vi "pickDefensiveTeam.vi"(0 "DefensiveTeam in":refnum<class "Ally.lvclass">, 1 "BallRef":refnum<class "Ball.lvclass">, 5 "KeeperTeam":refnum<class "Ally.lvclass">, 7 "OffensiveTeam":refnum<class "Ally.lvclass">, 9 "RobotRef in":refnum<class "Robot.lvclass">[](array[class]), 11 "error in (no error)":errorcluster, 12 "number_of_robots":i32, 13 "AllyTeamArray":T1[](array[typedef])) -> (4 "DefensiveTeam out":refnum<class "Ally.lvclass">, 8 "RobotRef":refnum<class "Robot.lvclass">[](array[class]), 15 "error out":errorcluster)   [LabVIEW 2023, in "Ally.lvclass"]
uses:
  Ally.lvclass
  Robot_class/Robot.lvclass
  Ball_class/Ball.lvclass
  Controls/AllyTeam.ctl
  Team_class/KeeperPlay.ctl
  Team_class/OffensivePlay.ctl
  Team_class/Team.lvclass/Team.ctl
  Robot_class/Robot.lvclass/Robot.ctl
  Utilities_class/Utilities.lvclass
  Robot_class/Read id.vi
  Team_class/Write RobotRef.vi
  Team_class/Read OffensivePlay.vi
  Team_class/Read RobotRef.vi
  Team_class/Read KeeperPlay.vi
  Team_class/Read DefensivePlay.vi
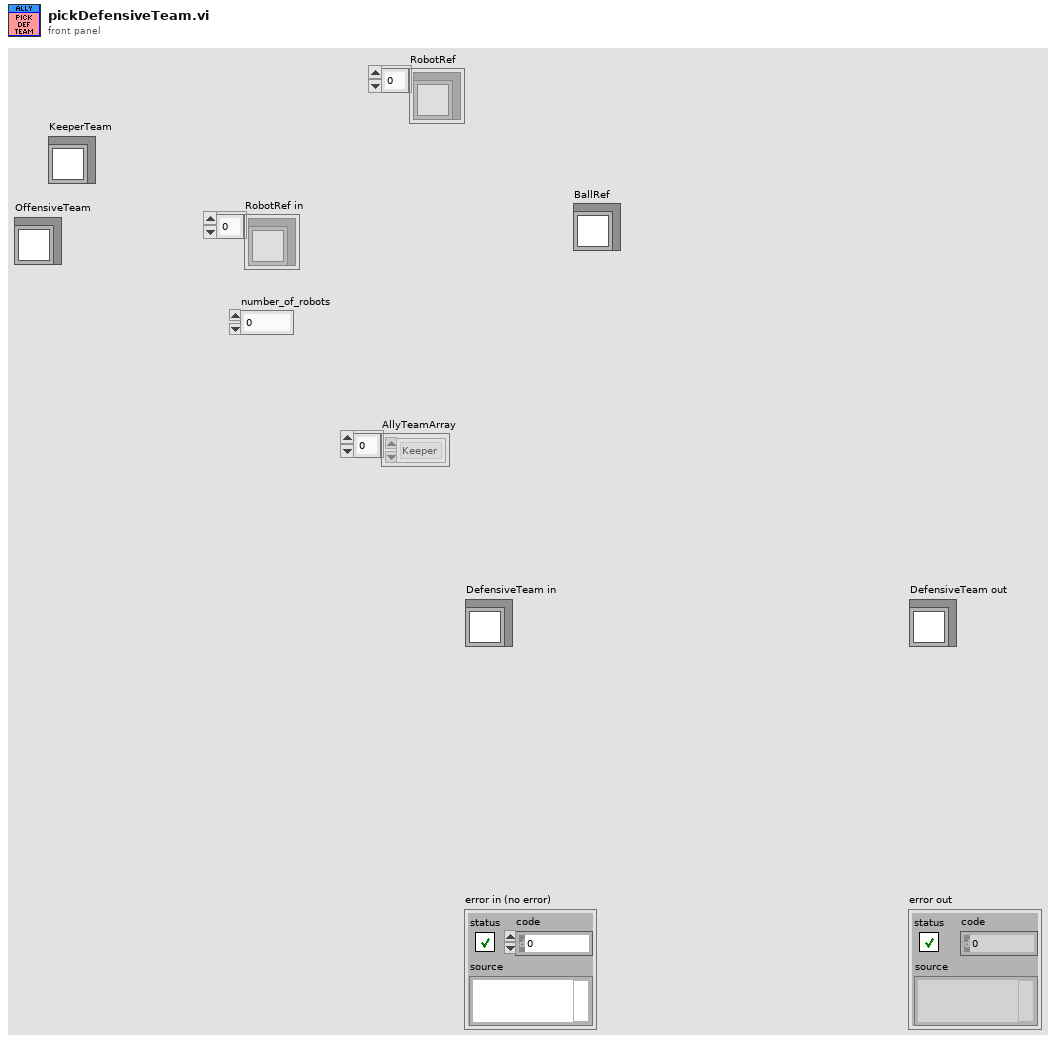
[diagram p1: front panel]
types:
  T1 = typedef "AllyTeam.ctl" = enum16{"Keeper", "Defender", "Attacker"}
  T2 = typedef "OffensivePlay.ctl" = enum16{"5RobotsPassGamePlay", "5PreparePassGame", "5RobotsKeeperGame", "KeeperPassToStriker", "5RobotsNormalGamePlay", "PrepareKeeperPass", "ACBPass", "ABCPass", "PrepareTriplePass", "TableWithStriker", "TableWith2ndStrikerPlay", "PrepareDoublePass", "PrepareRollToPass", "SimplePass", "PreparePass", "PassToStriker", "BallOutOfField", "PassTo2ndStriker", "StopOffensive", "Prepare Penalty Enemy", "EnemyPossessionAtEnemyField", "EnemyPossesionAtOurField", "TestPlay", "PreparePenaltyAlly", "KickPenaltyAlly", "PrepareKickoffAlly", "PrepareKickoffEnemy", "IndirectEnemy", "DirectEnemy", "PreparePassInGame1", "NormalGame", "DirectKick", "Pass", "Halt", "Timeout", "PassPlay", "PenaltyEnemy"}
  T3 = typedef "KeeperPlay.ctl" = enum16{"SimpleBallPlacementAlly", "BallPlacementAlly", "BallPlacementEnemy", "ZigZag", "Goto", "NormalGame", "KeeperPlay", "Halt", "Timeout", "PenaltyEnemy", "TestPlay"}
  T4 = typedef "DefensivePlay.ctl" = enum16{"NormalDefensiveWithDuelist", "NormalDefensive", "TestPlay", "Halt", "Timeout", "PenaltyEnemy", "PenaltyAlly"}
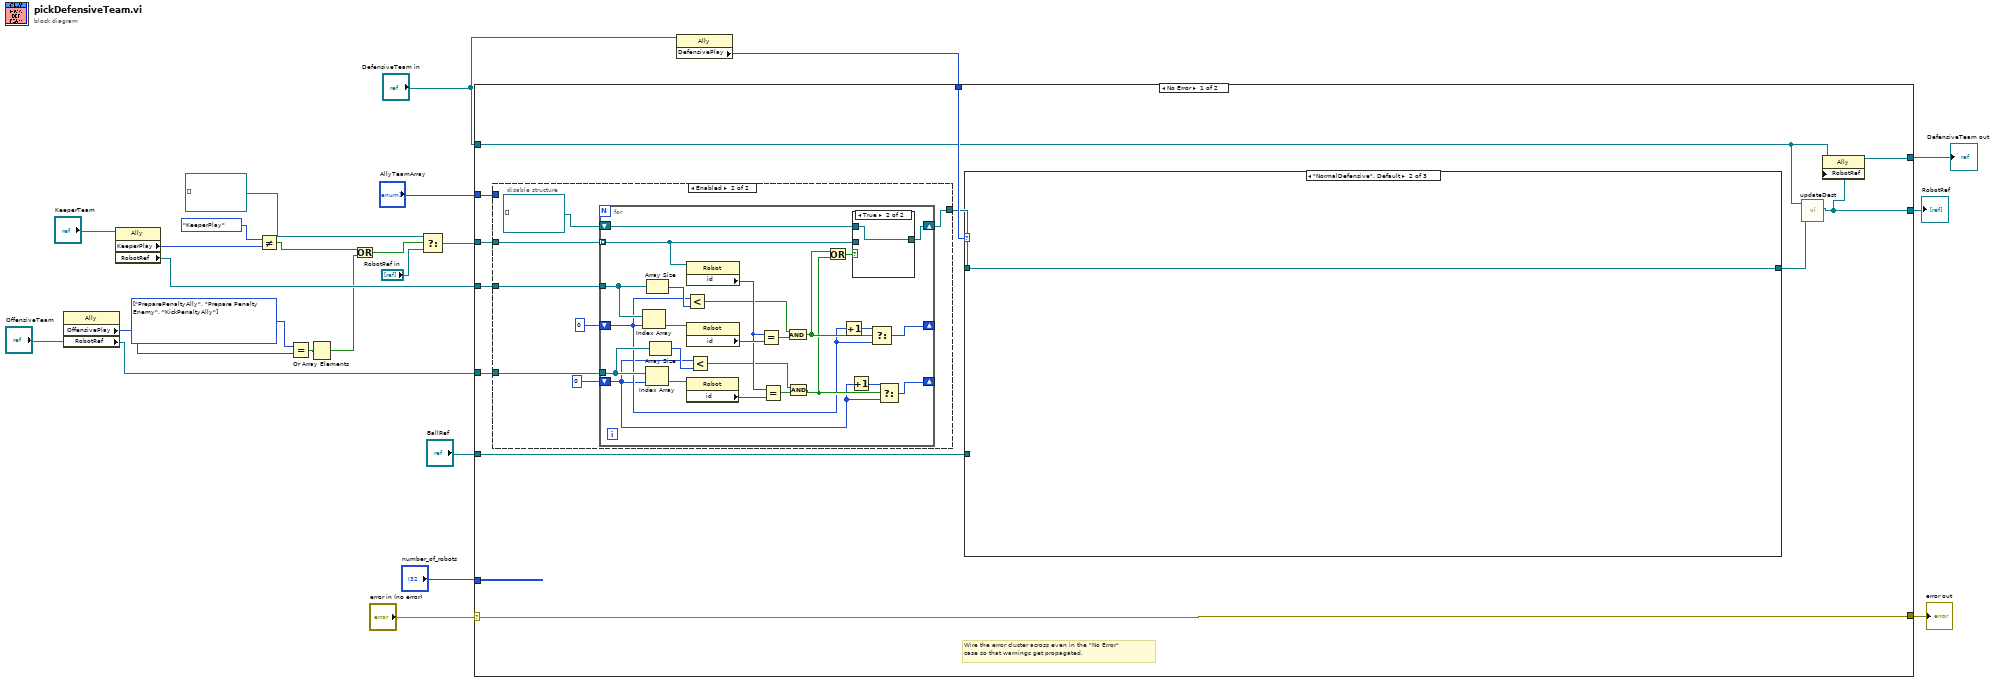
[diagram p0: block diagram]
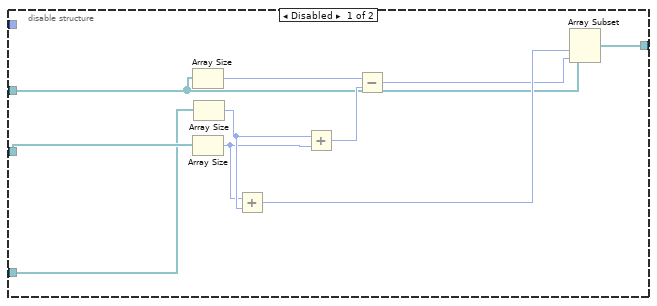
[diagram p2: hidden frame]
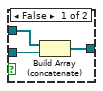
[diagram p3: hidden frame]
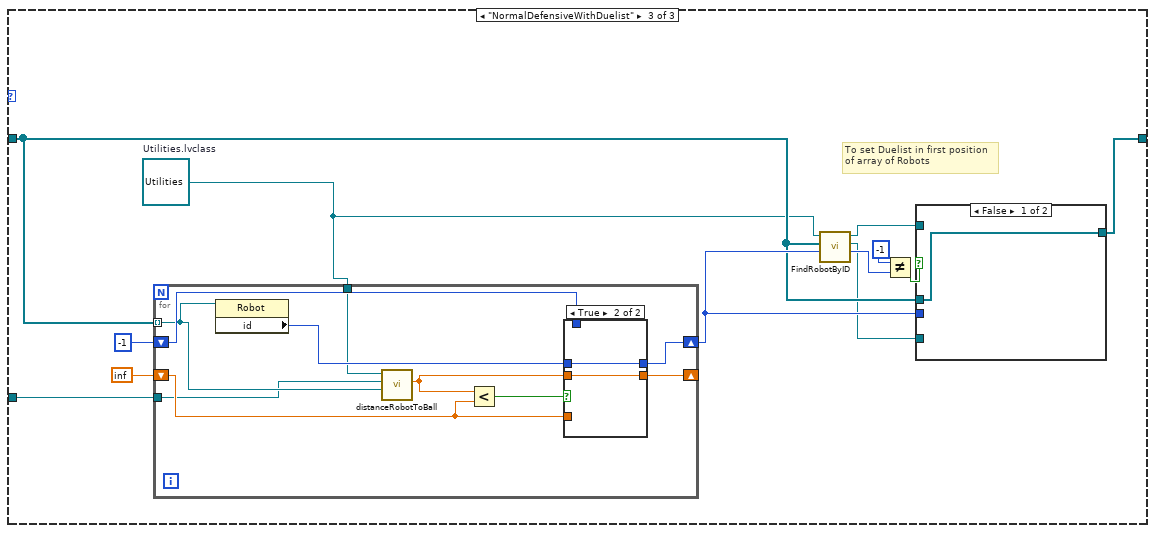
[diagram p5: hidden frame]
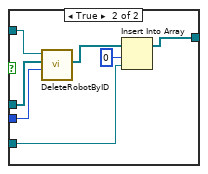
[diagram p6: hidden frame]
diagram:
  w5 = T2[] [enum."PreparePenaltyAlly", enum."Prepare Penalty Enemy", enum."KickPenaltyAlly"] items=["5RobotsPassGamePlay", "5PreparePassGame", "5RobotsKeeperGame", "KeeperPassToStriker", "5RobotsNormalGamePlay", "PrepareKeeperPass", "ACBPass", "ABCPass", "PrepareTriplePass", "TableWithStriker", "TableWith2ndStrikerPlay", "PrepareDoublePass", "PrepareRollToPass", "SimplePass", "PreparePass", "PassToStriker", "BallOutOfField", "PassTo2ndStriker", "StopOffensive", "Prepare Penalty Enemy", "EnemyPossessionAtEnemyField", "EnemyPossesionAtOurField", "TestPlay", "PreparePenaltyAlly", "KickPenaltyAlly", "PrepareKickoffAlly", "PrepareKickoffEnemy", "IndirectEnemy", "DirectEnemy", "PreparePassInGame1", "NormalGame", "DirectKick", "Pass", "Halt", "Timeout", "PassPlay", "PenaltyEnemy"] ("x")
  n1 = property class="Ally"(reference="OffensiveTeam") -> ("OffensivePlay"=w6:T2, "RobotRef"=w16:refnum<class "Robot.lvclass">[])  [unwired: 1 in, 2 out]
  n2 = property class="Ally"(reference="KeeperTeam") -> ("KeeperPlay"=w8:T3, "RobotRef"=w22:refnum<class "Robot.lvclass">[])  [unwired: 1 in, 2 out]
  n3 = Not Equal?(x=KeeperPlay."KeeperPlay" ("y"), y=w8) -> (x != y?=w4:bool)
  n4 = Equal?(x=w5, y=w6) -> (x = y?=w2:bool[])
  n5 = Or Array Elements(Boolean array=w2) -> (logical OR=w1:bool)
  n6 = Or(x=w4, y=w1) -> (x .or. y?=w3:bool)
  n7 = Select(t=refnum<class "Robot.lvclass">[] [], s=w3, f="RobotRef in") -> (s? t:f=w10:refnum<class "Robot.lvclass">[])
  n8 = property class="Ally"(reference="DefensiveTeam in") -> ("DefensivePlay"=w14:T4)  [unwired: 1 in, 2 out]
  n9 = case shown="No Error" "error in (no error)" {
    selector: "error in (no error)" -> [w36 w120]
    tunnel: [w36 w120] -> w18
    tunnel: [w35 w119] -> w19
    tunnel: "DefensiveTeam in" -> [w27 w119]
    tunnel: w10 -> [w30 _]
    tunnel: "number_of_robots" -> [_ _]
    tunnel: w22 -> [w34 _]
    tunnel: [w28 _] -> w21
    tunnel: w16 -> [w33 _]
    tunnel: w14 -> [w32 _]
    tunnel: "BallRef" -> [w26 _]
    tunnel: "AllyTeamArray" -> [w25 _]
    frame No Error {
      # "Wire the error cluster across even in the \"No Error\"\ncase so that warnings get propagated."
      n10 = disable-structure shown="Enabled" {
        disable-tunnel: w34 -> [w46 w50]
        disable-tunnel: w33 -> [w45 w49]
        disable-tunnel: [w43 w51] -> w31
        disable-tunnel: w30 -> [w39 w53]
        disable-tunnel: w25 -> [_ _]
        frame Disabled {
          n11 = Array Size(array=w39) -> (size(s)=w38:i32)
          n12 = Array Size(array=w46) -> (size(s)=w41:i32)
          n13 = Array Size(array=w45) -> (size(s)=w42:i32)
          n14 = Add(x=w41, y=w42) -> (x+y=w44:i32)
          n15 = Add(x=w42, y=w41) -> (x+y=w40:i32)
          n16 = Subtract(x=w38, y=w40) -> (x-y=w37:i32)
          n17 = Array Subset(array=w39, index=w44, length=w37) -> (w43:refnum<class "Robot.lvclass">[])
        }
        frame Enabled {
          n18 = for {
            tunnel: w53 -> [w76] mode=indexing
            shift-right: [w77] -> w51
            shift-left: refnum<class "Robot.lvclass">[] [] ("Array") -> [w78]
            tunnel: w49 -> [w58]
            tunnel: w50 -> [w67]
            shift-right: [w69] -> _
            shift-left: 0 -> [w54]
            shift-right: [w68] -> _
            shift-left: 0 -> [w56]
            n19 = Index Array(array=w67, index=w56) -> (element=w75:refnum<class "Robot.lvclass">)
            n20 = Index Array(array=w58, index=w54) -> (element=w74:refnum<class "Robot.lvclass">)
            n21 = Array Size(array=w67) -> (size(s)=w66:i32)
            n22 = Array Size(array=w58) -> (size(s)=w60:i32)
            n23 = Less?(x=w56, y=w66) -> (x < y?=w64:bool)
            n24 = property class="Robot"(reference=w74) -> ("id"=w71:i32)  [unwired: 1 in, 2 out]
            n25 = property class="Robot"(reference=w76) -> ("id"=w72:i32)  [unwired: 1 in, 2 out]
            n26 = property class="Robot"(reference=w75) -> ("id"=w73:i32)  [unwired: 1 in, 2 out]
            n27 = Less?(x=w54, y=w60) -> (x < y?=w59:bool)
            n28 = Equal?(x=w72, y=w73) -> (x = y?=w65:bool)
            n29 = Equal?(x=w72, y=w71) -> (x = y?=w62:bool)
            n30 = And(x=w64, y=w65) -> (x .and. y?=w63:bool)
            n31 = And(x=w59, y=w62) -> (x .and. y?=w61:bool)
            n32 = Or(x=w63, y=w61) -> (x .or. y?=w70:bool)
            n33 = Increment(x=w56) -> (x+1=w57:i32)
            n34 = Increment(x=w54) -> (x+1=w55:i32)
            n35 = case shown="True" w70 {
              tunnel: w78 -> [w81 w82]
              tunnel: [w80 w82] -> w77
              tunnel: w76 -> [w79 _]
              frame False {
                n36 = Build Array (concatenate)(w81, w79) -> (w80:refnum<class "Robot.lvclass">[])
              }
              frame True {
              }
            }
            n37 = Select(t=w57, s=w63, f=w56) -> (s? t:f=w68:i32)
            n38 = Select(t=w55, s=w61, f=w54) -> (s? t:f=w69:i32)
          }
        }
      }
      n39 = case shown="\"NormalDefensive\", Default" w32 {
        tunnel: [w83 w84 w92] -> w29
        tunnel: w31 -> [w83 w84 w91]
        tunnel: w26 -> [_ _ w85]
        frame "TestPlay" {
          # "Aqui entra a lógica para\nreeordenar o team de acordo \ncom quem deve assumir cada\nrole"
        }
        frame "NormalDefensive", Default {
        }
        frame "NormalDefensiveWithDuelist" {
          w90 = refnum<class "Utilities.lvclass"> refnum  # Utilities.lvclass
          # "To set Duelist in first position\nof array of Robots"
          n40 = for {
            tunnel: w91 -> [w106] mode=indexing
            shift-right: [w113] -> w95
            shift-left: -1 ("id") -> [w110]
            shift-right: [w111] -> _
            shift-left: inf -> [w109]
            tunnel: w90 -> [w108]
            tunnel: w85 -> [w105]
            n41 = property class="Robot"(reference=w106) -> ("id"=w112:i32)  [unwired: 1 in, 2 out]
            n42 = call "distanceRobotToBall.vi"("Robot"=w106, "Ball"=w105, "Utilities in"=w108) -> ("Distance Robot To Ball"=w107:dbl)  [unwired: 6 in, 2 out]
            n43 = Less?(x=w107, y=w109) -> (x < y?=w114:bool)
            n44 = case shown="True" w114 {
              tunnel: [w116 w118] -> w113
              tunnel: w112 -> [_ w118]
              tunnel: [w115 w117] -> w111
              tunnel: w107 -> [_ w117]
              tunnel: w110 -> [w116 _]
              tunnel: w109 -> [w115 _]
              frame False {
              }
              frame True {
              }
            }
          }
          n45 = call "FindRobotByID.vi"("id"=w95, "RobotRef"=w91, "Utilities in"=w90) -> ("index"=w89:i32, "Robot"=w86:refnum<class "Robot.lvclass">, "Utilities out"=w94:refnum<class "Utilities.lvclass">)  [unwired: 5 in, 1 out]
          n46 = Not Equal?(x=-1, y=w89) -> (x != y?=w87:bool)
          n47 = case shown="False" w87 {
            tunnel: w95 -> [_ w102]
            tunnel: w94 -> [_ w104]
            tunnel: [w97 w98] -> w92
            tunnel: w91 -> [w97 w103]
            tunnel: w86 -> [_ w100]
            frame False {
            }
            frame True {
              n48 = call "DeleteRobotByID.vi"("id"=w102, "RobotRef"=w103, "Utilities in"=w104) -> ("RobotRef out"=w101:refnum<class "Robot.lvclass">[])  [unwired: 6 in, 2 out]
              n49 = Insert Into Array(array=w101, index=0, new element=w100) -> (w98:refnum<class "Robot.lvclass">[])
            }
          }
        }
      }
      n50 = call "updateDest.vi"("NewAllyRobots"=w29, "LastAlly"=w27) -> ("NewAllyRobotsUpdated"=w28:refnum<class "Robot.lvclass">[])  [unwired: 7 in, 2 out]
      n51 = property class="Ally"(reference=w27, "RobotRef"=w28) -> (reference out=w35:refnum<class "Ally.lvclass">)  [unwired: 1 in, 1 out]
    }
    frame Error {
    }
  }
  "error out" <- w18
  "DefensiveTeam out" <- w19
  "RobotRef" <- w21
